vi "getConnectionPoints.vi"(0 "reference":refnum<class "StateTransitionEdge.lvclass">, 5 "error in (no error)":errorcluster) -> (14 "reference out":refnum<class "StateTransitionEdge.lvclass">, 15 "line":T1[](array[typedef]) {"y" format="%.2f"; "x" format="%.2f"}, 19 "error out":errorcluster)   [LabVIEW 2016, in "StateTransitionEdge.lvclass"]
doc: "public Line2D getConnectionPoints()"
uses:
  <resource>/Framework/Providers/Open_GDS/UML/StateTransitionEdge_class/StateTransitionEdge.lvclass
  C:/Program Files (x86)/National Instruments/LabVIEW 2016/resource/Framework/Providers/Open_GDS/UML/ClassRelationshipEdge_class/ClassRelationshipEdge.lvclass
  C:/Program Files (x86)/National Instruments/LabVIEW 2016/resource/Framework/Providers/Open_GDS/UML/AbstractEdge_class/AbstractEdge.lvclass
  <resource>/Framework/Providers/Open_GDS/UML/General/Point/Point Point2D.ctl
  <resource>/Framework/Providers/Open_GDS/UML/BentStyle_class/BentStyle.lvclass
  <resource>/Framework/Providers/Open_GDS/UML/ClassRelationshipEdge_class/ClassRelationshipEdge.lvclass
  <resource>/Framework/Providers/Open_GDS/UML/AbstractNode_class/AbstractNode.lvclass
  <resource>/Framework/Providers/Open_GDS/UML/Direction_class/Direction.lvclass
  <resource>/Framework/Providers/Open_GDS/UML/AbstractEdge_class/AbstractEdge.lvclass
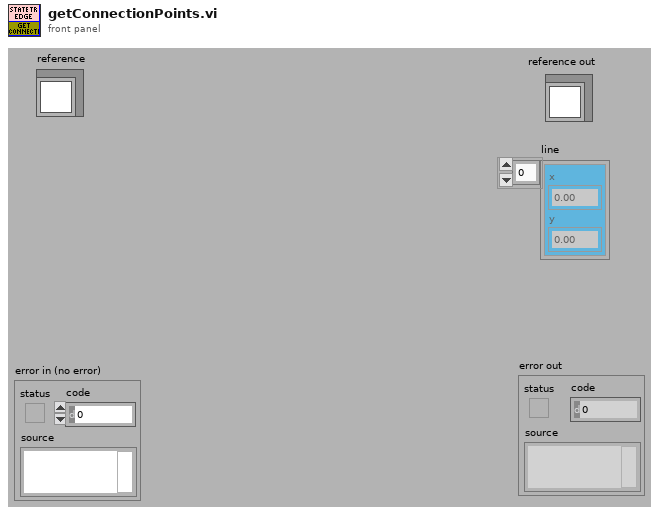
[diagram p1: front panel]
types:
  T1 = typedef "Point Point2D.ctl" = cluster{"x":dbl, "y":dbl}
  T2 = typedef "ClassRelationshipEdge.lvclass/ObjectAttributes.ctl" = cluster{"bentStyleRef":refnum<class "BentStyle.lvclass">, "startConnectionOffset":cluster{"x":i32, "y":i32}, "endConnectionOffset":cluster{"x":i32, "y":i32}, "MidLineOffset":cluster{"x":i32, "y":i32}, "DepClass":T3}
  T3 = typedef "ReversedEngineering_ViDependencyDetailsType.ctl" = cluster{"ThisVIs/Ctls":path[], "Dependent_VIs/Ctls":path[]}
  T4 = typedef "AbstractEdge.lvclass/ObjectAttributes.ctl" = cluster{"start":refnum<class "AbstractNode.lvclass">, "end":refnum<class "AbstractNode.lvclass">}
  T5 = typedef "BentStyle.lvclass/BentStyleType.ctl" = enum16{"STRAIGHT", "HV", "VH", "HVH", "VHV", "ARC"}
  T6 = typedef "StateTransitionEdge.lvclass/ObjectAttributes.ctl" = cluster{"angle":dbl}
  T7 = typedef "Rectangle Rectangle2D.ctl" = cluster{"x":dbl, "y":dbl, "width":dbl, "height":dbl}
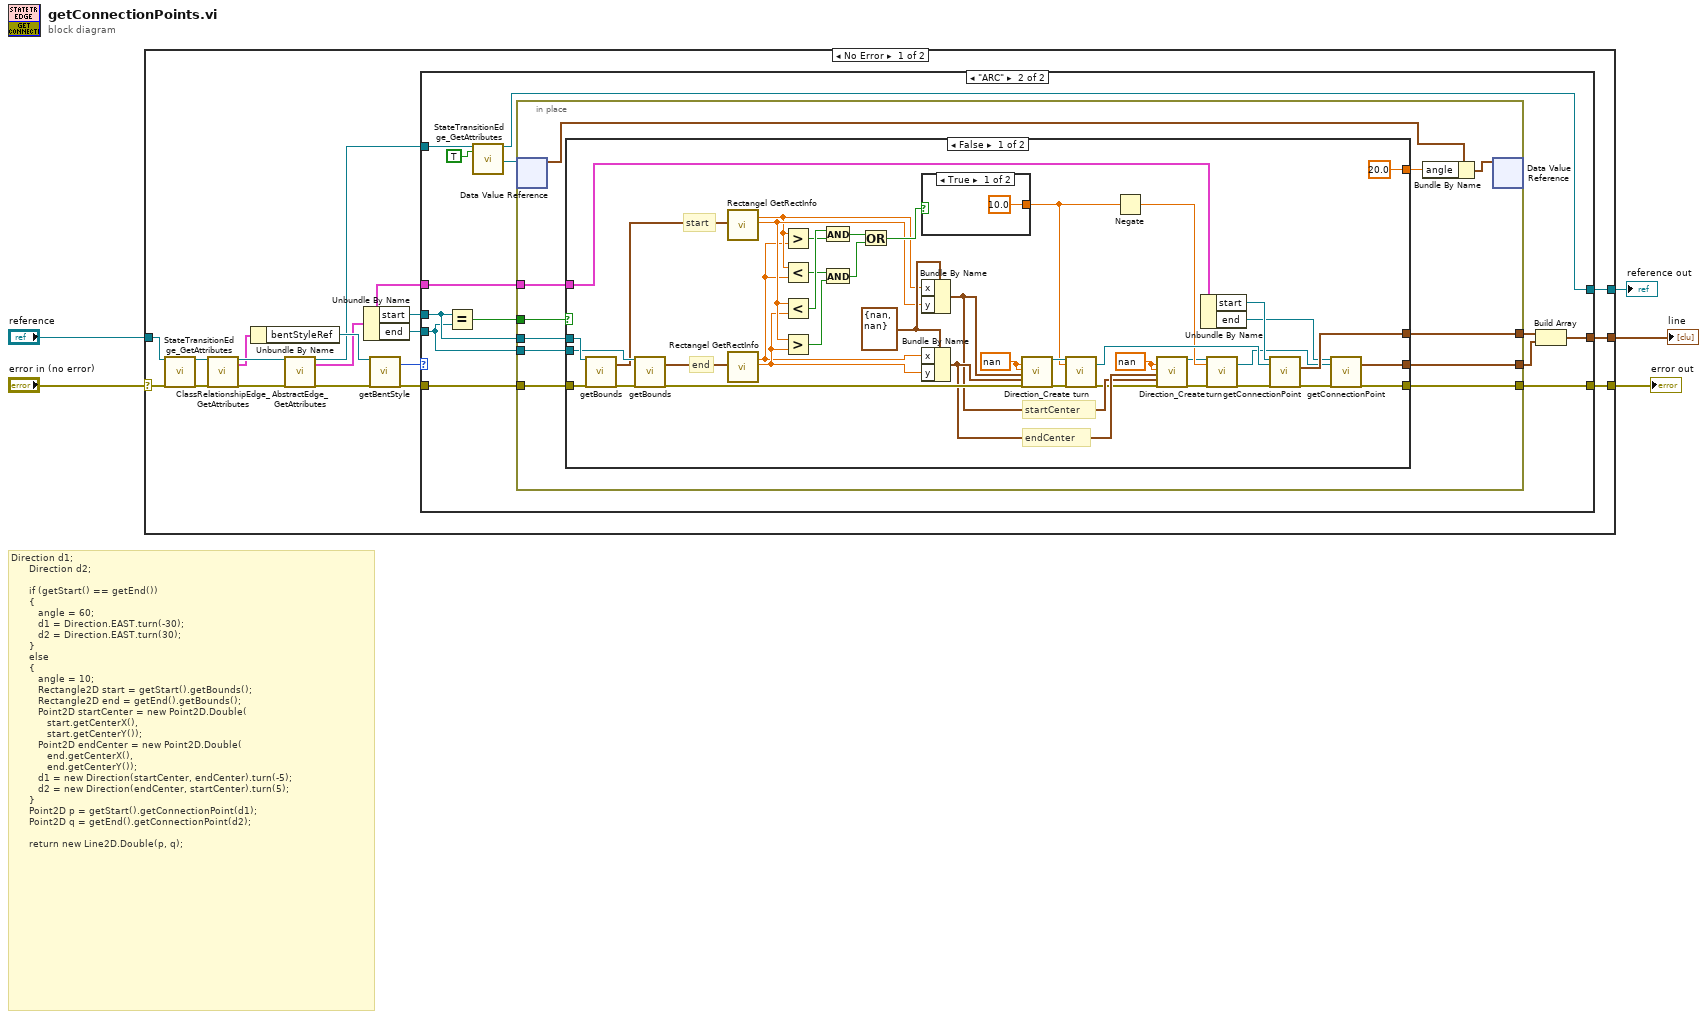
[diagram p0: block diagram]
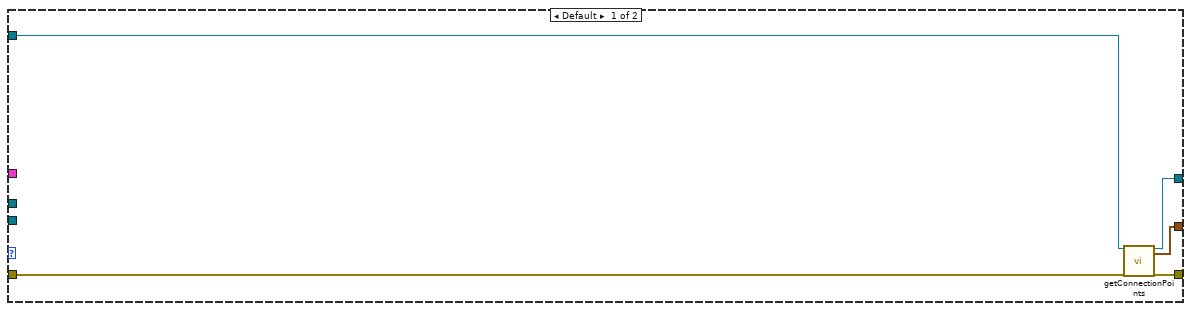
[diagram p2: hidden frame]
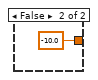
[diagram p3: hidden frame]
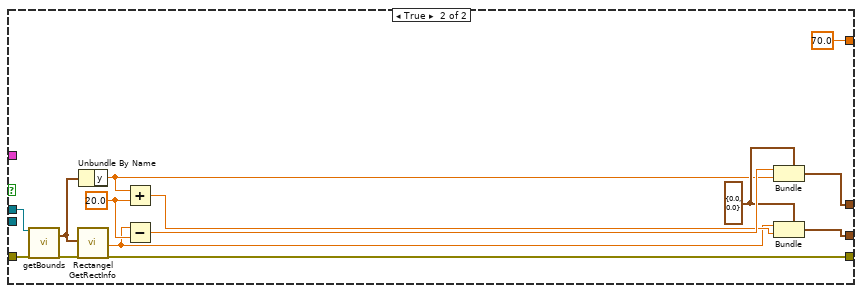
[diagram p4: hidden frame]
diagram:
  # "Direction d1;\n      Direction d2;\n\n      if (getStart() == getEnd())\n      {\n         angle = 60;\n         d1 = Direction.EAST.turn(-30);\n         d2 = Direction.EAST.turn(30);\n      }\n      else\n      {\n         angle = 10;\n         Rectangle2D start = getStart().getBounds();\n         Rectangle2D end = getEnd().getBounds();\n         Point2D startCenter = new Point2D.Double(\n            start.getCenterX(),\n            start.getCenterY());\n         Point2D endCenter = new Point2D.Double(\n            end.getCenterX(),\n            end.getCenterY());\n         d1 = new Direction(startCenter, endCenter).turn(-5);\n         d2 = new Direction(endCenter, startCenter).turn(5);\n      }\n      Point2D p = getStart().getConnectionPoint(d1);\n      Point2D q = getEnd().getConnectionPoint(d2);\n\n      return new Line2D.Double(p, q);"
  n1 = case shown="No Error" "error in (no error)" {
    selector: "error in (no error)" -> [w16 w110]
    tunnel: "reference" -> [w22 w111]
    tunnel: [w21 w110] -> w4
    tunnel: [w18 w111] -> w3
    tunnel: [w23 _] -> w1
    frame No Error {
      n2 = call <resource>:"StateTransitionEdge_GetAttributes.vi"("reference in"=w22, "error in (no error)"=w16) -> ("reference out"=w13:refnum<class "StateTransitionEdge.lvclass">, "error out"=w12:errorcluster)  [unwired: 1 in, 15 out]
      n3 = call <resource>:"ClassRelationshipEdge_GetAttributes.vi"("reference in"=w13, "error in (no error)"=w12) -> ("reference out"=w11:refnum<class "StateTransitionEdge.lvclass">, "Data"=w7:T2, "error out"=w10:errorcluster)  [unwired: 14 in, 1 out]
      n4 = Unbundle By Name(w7) -> ("bentStyleRef"=w17:refnum<class "BentStyle.lvclass">)
      n5 = call <resource>:"AbstractEdge_GetAttributes.vi"("reference in"=w11, "error in (no error)"=w10) -> ("reference out"=w8:refnum<class "StateTransitionEdge.lvclass">, "Data"=w6:T4, "error out"=w9:errorcluster)  [unwired: 14 in, 1 out]
      n6 = Unbundle By Name(w6) -> ("start"=w20:refnum<class "AbstractNode.lvclass">, "end"=w19:refnum<class "AbstractNode.lvclass">)
      n7 = call-dynamic "getBentStyle.vi"("reference"=w17, "error in (no error)"=w9) -> ("bentStyle"=w14:T5, "error out"=w15:errorcluster)  [unwired: 15 in, 1 out]
      n8 = case shown="\"ARC\"" w14 {
        tunnel: [w26 w41] -> w23
        tunnel: [w25 w30] -> w21
        tunnel: w20 -> [_ w35]
        tunnel: w19 -> [_ w34]
        tunnel: [w27 w40] -> w18
        tunnel: w8 -> [w28 w39]
        tunnel: w15 -> [w24 w33]
        tunnel: w6 -> [_ w29]
        frame Default {
          n9 = call-parent "getConnectionPoints.vi"("reference"=w28, "error in (no error)"=w24) -> ("reference out"=w27:refnum<class "StateTransitionEdge.lvclass">, "line"=w26:T1[], "error out"=w25:errorcluster)  [unwired: 15 in]
        }
        frame "ARC" {
          n10 = Equal?(x=w35, y=w34) -> (x = y?=w36:bool)
          n11 = call <resource>:"StateTransitionEdge_GetAttributes.vi"("reference in"=w39, "OnlyGetDvrReference(False)"=TRUE) -> ("reference out"=w40:refnum<class "StateTransitionEdge.lvclass">, "DataRef"=w37:refnum<data-value>)  [unwired: 14 in, 2 out]
          n12 = in-place {
            in-place-border: w36 -> [w49]
            in-place-border: w35 -> [w48]
            in-place-border: w34 -> [w47]
            in-place-border: w33 -> [w46]
            in-place-border: [w45] -> w32
            in-place-border: [w44] -> w31
            in-place-border: [w43] -> w30
            in-place-border: w29 -> [w42]
            n13 = in-place-dvr #1(w37) -> (w52:T6)  [unwired: 1 out]
            n14 = case shown="False" w49 {
              tunnel: [w92 w101] -> w45
              tunnel: [w89 w100] -> w44
              tunnel: [w56 w99] -> w43
              tunnel: w48 -> [w86 w107]
              tunnel: w47 -> [w85 _]
              tunnel: [20.0 ("angle") 70.0 ("angle")] -> w51
              tunnel: w46 -> [w83 w108]
              tunnel: w42 -> [w53 _]
              frame False {
                w79 = T1 {"x"=nan, "y"=nan} ("p1")
                w57 = nan ("dx")
                w58 = nan ("dx")
                # "endCenter"
                # "startCenter"
                # "end"
                # "start"
                n15 = call-dynamic "getBounds.vi"("reference"=w86, "error in (no error)"=w83) -> ("bounds"=w81:T7, "error out"=w80:errorcluster)  [unwired: 15 in, 1 out]
                n16 = call-dynamic "getBounds.vi"("reference"=w85, "error in (no error)"=w80) -> ("bounds"=w82:T7, "error out"=w72:errorcluster)  [unwired: 15 in, 1 out]
                n17 = call <resource>:"Rectangel GetRectInfo.vi"("bounds"=w81) -> ("centerX"=w60:dbl, "centerY"=w62:dbl)  [unwired: 1 in, 16 out]
                n18 = call <resource>:"Rectangel GetRectInfo.vi"("bounds"=w82) -> ("centerX"=w59:dbl, "centerY"=w61:dbl)  [unwired: 1 in, 16 out]
                n19 = Greater?(x=w60, y=w59) -> (0:w67:bool)
                n20 = Less?(x=w60, y=w59) -> (x < y?=w66:bool)
                n21 = Less?(x=w62, y=w61) -> (x < y?=w68:bool)
                n22 = Greater?(x=w62, y=w61) -> (0:w65:bool)
                n23 = And(x=w68, y=w67) -> (x .and. y?=w69:bool)
                n24 = And(x=w66, y=w65) -> (x .and. y?=w64:bool)
                n25 = Or(x=w69, y=w64) -> (x .or. y?=w63:bool)
                n26 = case shown="True" w63 {
                  tunnel: [10.0 ("angle") -10.0 ("angle")] -> w76
                  frame True {
                  }
                  frame False {
                  }
                }
                n27 = Bundle By Name(cluster=w79, "x"=w60, "y"=w62) -> (w70:T1)
                n28 = Bundle By Name(cluster=w79, "x"=w59, "y"=w61) -> (w71:T1)
                n29 = call <resource>:"Direction_Create.vi"("dx"=w57, "dy"=w57, "p1"=w70, "p2"=w71, "error in (no error)"=w72) -> ("reference out"=w78:refnum<class "Direction.lvclass">, "error out"=w77:errorcluster)  [unwired: 13 in]
                n30 = call <resource>:"turn.vi"("reference"=w78, "angle"=w76, "error in (no error)"=w77) -> ("turnedDirection"=w88:refnum<class "Direction.lvclass">, "error out"=w55:errorcluster)  [unwired: 15 out]
                n31 = Negate(x=w76) -> (-x=w74:dbl)
                n32 = call <resource>:"Direction_Create.vi"("dx"=w58, "dy"=w58, "p1"=w71, "p2"=w70, "error in (no error)"=w55) -> ("reference out"=w73:refnum<class "Direction.lvclass">, "error out"=w75:errorcluster)  [unwired: 13 in]
                n33 = Unbundle By Name(w53) -> ("start"=w93:refnum<class "AbstractNode.lvclass">, "end"=w91:refnum<class "AbstractNode.lvclass">)
                n34 = call <resource>:"turn.vi"("reference"=w73, "angle"=w74, "error in (no error)"=w75) -> ("turnedDirection"=w87:refnum<class "Direction.lvclass">, "error out"=w54:errorcluster)  [unwired: 15 out]
                n35 = call-dynamic "getConnectionPoint.vi"("reference"=w93, "direction"=w88, "error in (no error)"=w54) -> ("point2D"=w92:T1, "error out"=w90:errorcluster)  [unwired: 14 in, 1 out]
                n36 = call-dynamic "getConnectionPoint.vi"("reference"=w91, "direction"=w87, "error in (no error)"=w90) -> ("point2D"=w89:T1, "error out"=w56:errorcluster)  [unwired: 14 in, 1 out]
              }
              frame True {
                w103 = T1 {"x"=0.0, "y"=0.0} ("point2D")
                w105 = 20.0 ("y")
                n37 = call-dynamic "getBounds.vi"("reference"=w107, "error in (no error)"=w108) -> ("bounds"=w98:T7, "error out"=w106:errorcluster)  [unwired: 15 in, 1 out]
                n38 = call <resource>:"Rectangel GetRectInfo.vi"("bounds"=w98, "error in (no error)"=w106) -> ("maxX"=w97:dbl, "error out"=w99:errorcluster)  [unwired: 16 out]
                n39 = Unbundle By Name(w98) -> ("y"=w96:dbl)
                n40 = Add(x=w96, y=w105) -> (x+y=w102:dbl)
                n41 = Subtract(x=w97, y=w105) -> (x-y=w104:dbl)
                n42 = Bundle(cluster=w103, "x"=w104, "y"=w96) -> (w101:T1)
                n43 = Bundle(cluster=w103, "x"=w97, "y"=w102) -> (w100:T1)
              }
            }
            n44 = Bundle By Name(cluster=w52, "angle"=w51) -> (w50:T6)
            n45 = in-place-dvr #1(w50) -> ()  [unwired: 2 out]
          }
          n46 = Build Array(w32, w31) -> (w41:T1[])
        }
      }
    }
    frame Error {
    }
  }
  "reference out" <- w3
  "error out" <- w4
  "line" <- w1
